vi "SendPPMSCommand_Example.vi"() -> ()   [LabVIEW 2019]
panel:
  out "SendPPMSCommand Error 2":i32
  out "PpmsReply 2":string
  in  "PpmsCommand 2":string="DIGSET?"
  out "SendPPMSCommand Error":i32
  out "PpmsReply":string
  in  "PpmsCommand":string="DIGSET 1"
  in  "Remote":bool
  in  "IP Address":string="127.0.0.1"
  # "First Command/Reply"
  # "Second Command/Reply"
  # "Instrument Connection"
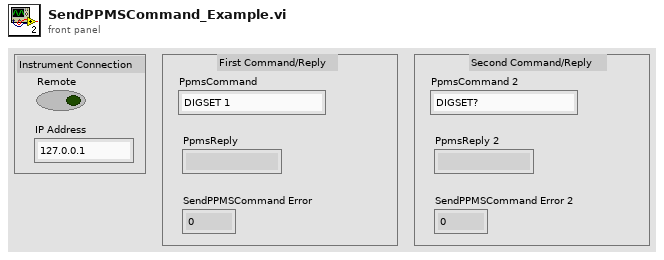
[diagram p1: front panel]
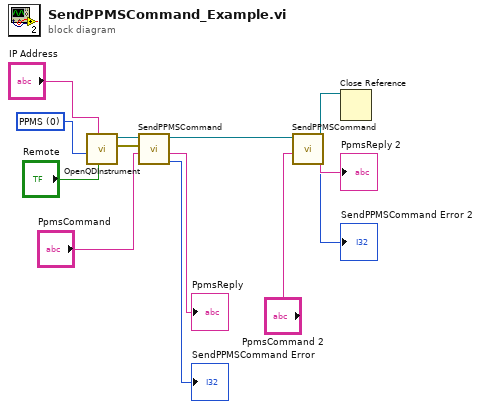
[diagram p0: block diagram]
diagram:
  w9 = 0 items=["PPMS", "VersaLab", "DynaCool", "SVSM"] ("Instrument Type")
  n1 = call "OpenQDInstrument.vi"("Remote"="Remote", "IP Address"="IP Address", "InstrumentType"=w9) -> ("error out"=w12:errorcluster, "Instrument Ref"=w13:refnum<k24>)  [unwired: 5 in]
  n2 = call "SendPPMSCommand.vi"("PpmsCommand"="PpmsCommand", "error in (no error)"=w12, "Instrument Ref In"=w13) -> ("SendPPMSCommand Error"=→"SendPPMSCommand Error":i32, "PpmsReply"=→"PpmsReply":string, "Instrument Ref Out"=w2:refnum<k24>)  [unwired: 4 in, 2 out]
  n3 = call "SendPPMSCommand.vi"("PpmsCommand"="PpmsCommand 2", "Instrument Ref In"=w2) -> ("SendPPMSCommand Error"=→"SendPPMSCommand Error 2":i32, "PpmsReply"=→"PpmsReply 2":string, "Instrument Ref Out"=w5:refnum<k24>)  [unwired: 5 in, 2 out]
  n4 = Close Reference(reference=w5) -> ()  [unwired: 1 in, 1 out]
